vi "校准数据全局变量.vi"() -> ()   [LabVIEW 2016]
panel:
  in  "CODMn曲线模型":T1(array[cluster]) {"r^2 2" format="%.7f"; "标定时间" format="%<%m/%d/%y %H:%M:%S>T"; "标样五校准时间" format="%<%m/%d/%y %H:%M:%S>T"; "标样四校准时间" format="%<%m/%d/%y %H:%M:%S>T"; "标样三校准时间" format="%<%m/%d/%y %H:%M:%S>T"; "标样二校准时间" format="%<%m/%d/%y %H:%M:%S>T"; "标样一校准时间" format="%<%m/%d/%y %H:%M:%S>T"; "r^2" format="%.7f"; "测量吸光度5" format="%#.6f"; "测量吸光度4" format="%#.6f"; "测量吸光度3" format="%#.6f"; "测量吸光度2" format="%#.6f"; "测量吸光度1" format="%#.6f"}
  # "校准时间"
  # "标液浓度"
  # "吸光值显示"
  # "标液一"
  # "标液二"
  # "标液三"
  # "零点"
  # "跨度"
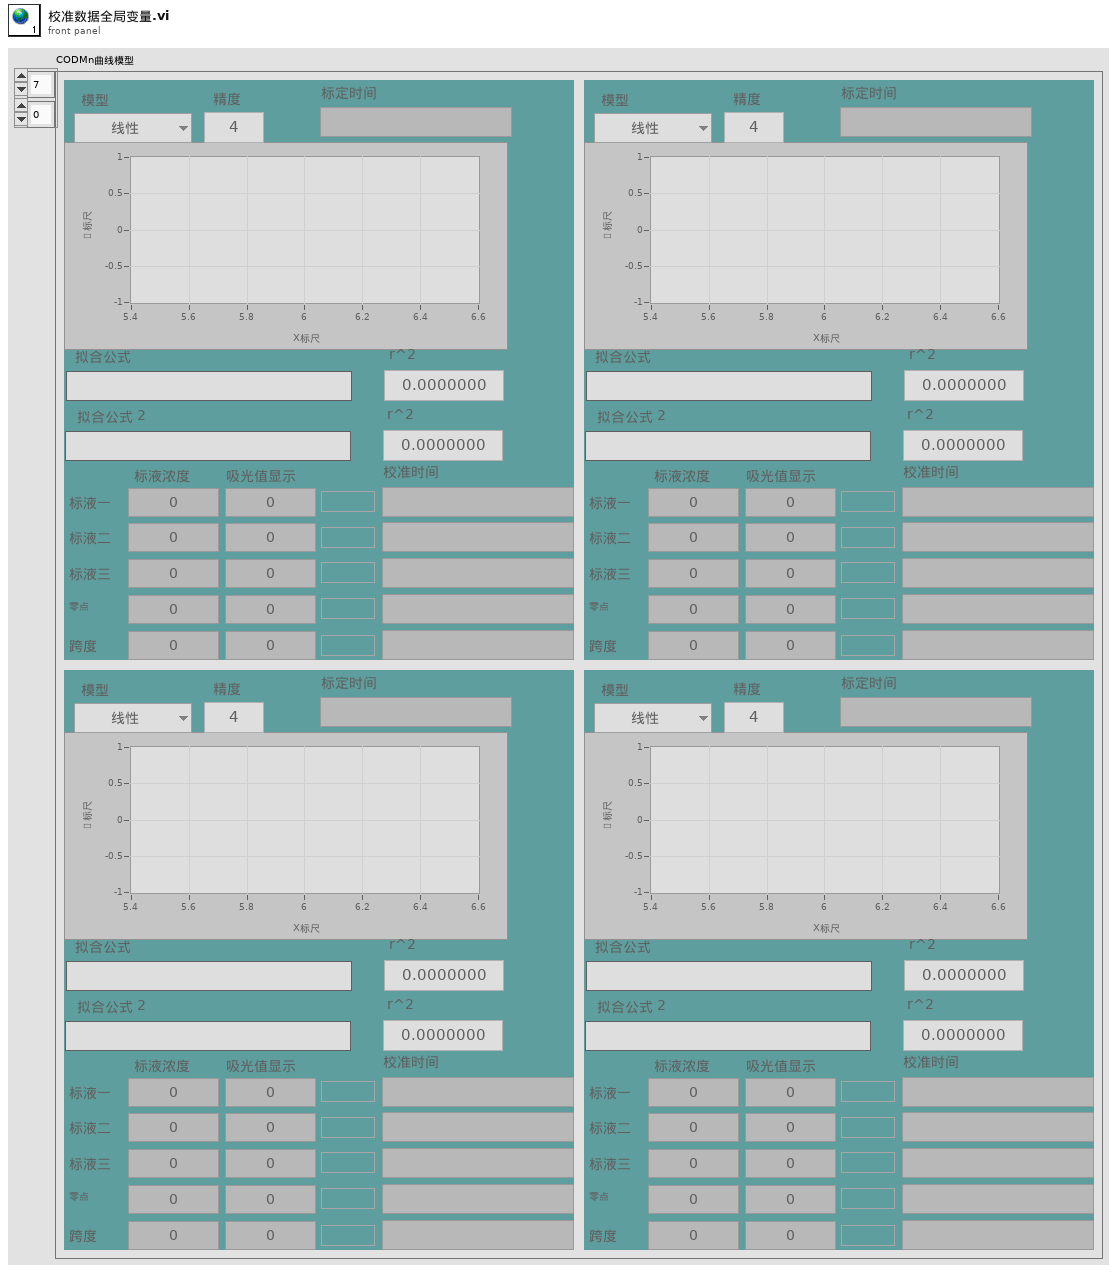
[diagram p1: front panel]
types:
  T1 = cluster{"标液浓度1":dbl, "测量吸光度1":dbl, "样品1启用":bool, "标液浓度2":dbl, "测量吸光度2":dbl, "样品2启用":bool, "标液浓度3":dbl, "测量吸光度3":dbl, "样品3启用":bool, "标液浓度4":dbl, "测量吸光度4":dbl, "样品4启用":bool, "标液浓度5":dbl, "测量吸光度5":dbl, "样品5启用":bool, "模型":enum32{"线性", "多项式", "折线"}, "精度":dbl, "XY图":cluster{"X Values":dbl[], "Y Values":dbl[]}[], "拟合公式":string, "r^2":dbl, "标样一校准时间":timestamp, "标样二校准时间":timestamp, "标样三校准时间":timestamp, "标样四校准时间":timestamp, "标样五校准时间":timestamp, "二次方程":cluster{"c":dbl, "x":dbl, "x^2":dbl}, "标定时间":timestamp, "拟合公式 2":string, "r^2 2":dbl}[][]
diagram:
